vi "Camera Dialog.vi"(8 "error in":errorcluster, 9 "Set Points":dbl[](array[numeric])=[1.0, 5.0, 1.0, 0.0]) -> (0 "error out":errorcluster, 1 "ROI":T3, 2 "Image Out":T1(plugin-control), 3 "Session out":T2="cam1")   [LabVIEW 2012]
uses:
  <vilib>/vision/driver/NI_Vision_Acquisition_Software.lvlib
  <vilib>/userdefined/High Color/IMAQdx.ctl
panel:
  in  "Tab Control":enum32{"Configure", "Help", "Advanced"}(tab)
  in  "Record images":bool
  out "Interface elevation":dbl
  in  "Image folder":path
  in  "Image Save Rate (s)":dbl=10.0 format="%#_5f"
  in  "Update Camera":bool
  in  "Camera Attributes In":string
  out "Camera Attributes":string
  out "Camera error out":errorcluster
  out "stop":bool
  in  "Cancel Button":bool
  in  "OK Button":bool
  # "Use the rectangle tool to define the region of interest where the floc water interface will appear.\nThe region of interest is saved in a configuration file.\n\nChoose a folder to save images during the experiment."
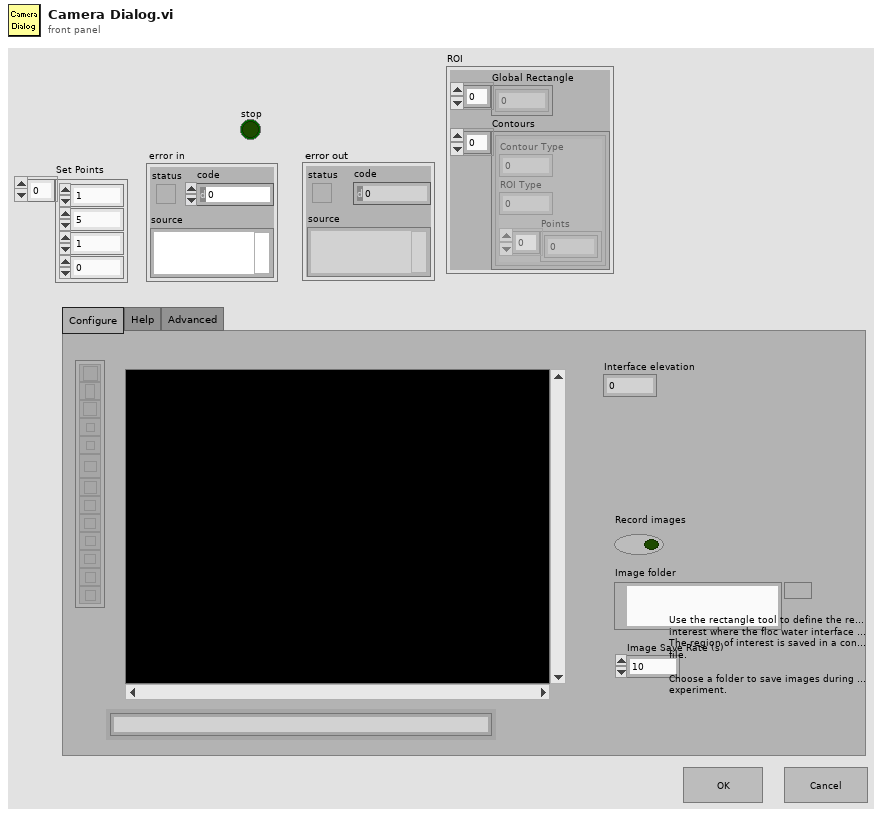
[diagram p1: front panel]
types:
  T1 = typedef "IMAQ Image.ctl" = refnum<image>
  T2 = typedef "IMAQdx.ctl" = refnum<k21>
  T3 = cluster{"Global Rectangle":i32[], "Contours":cluster{"Contour Type":u32, "ROI Type":u32, "Points":i32[]}[]}
  T4 = typedef "Image Type" = u32
  T5 = cluster{"Set Points[0]":dbl, "Set Points[1]":dbl, "Set Points[2]":dbl, "Set Points[3]":dbl}
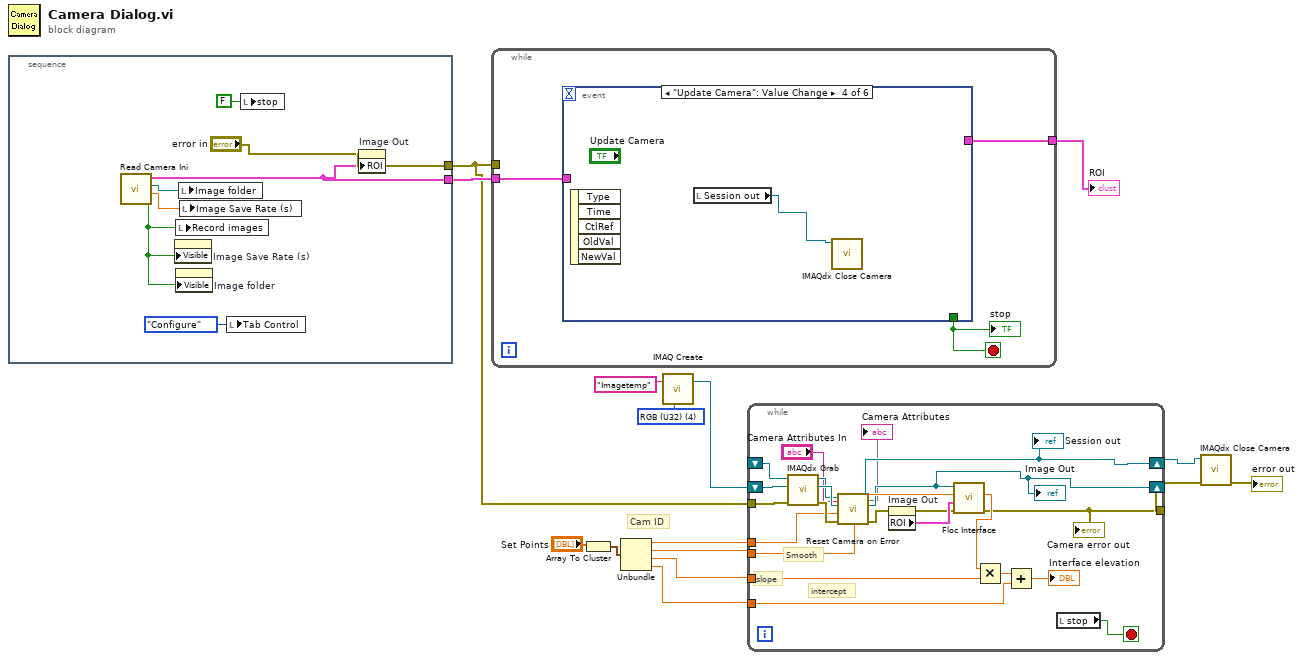
[diagram p0: block diagram]
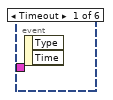
[diagram p2: hidden frame]
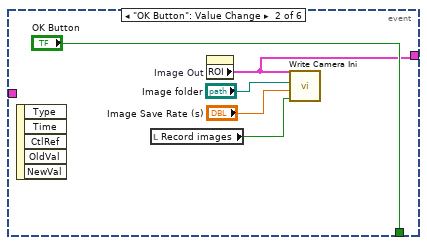
[diagram p3: hidden frame]
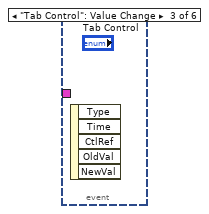
[diagram p4: hidden frame]
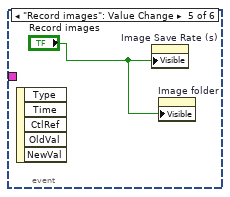
[diagram p5: hidden frame]
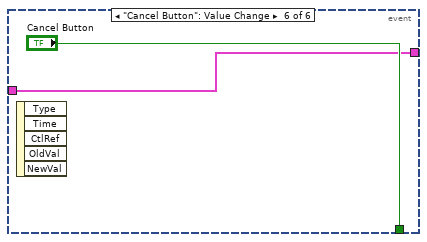
[diagram p6: hidden frame]
diagram:
  w8 = T4 4 items=["Grayscale (U8)", "Grayscale (I16)", "Grayscale (SGL)", "Complex (CSG)", "RGB (U32)", "HSL (U32)", "RGB (U64)", "Grayscale (U16)"] ("Image Type")
  # "Cam ID"
  n1 = stacked-sequence {
    tunnel: [w23] -> w1
    tunnel: [w21] -> w9
    frame #0 {
      n2 = call "Read Camera Ini.vi"() -> ("Record images"=w17:bool, "Image Save Rate (s)"=w18:dbl, "Image folder"=w19:path, "ROI"=w21:T3)  [unwired: 8 in]
      n3 = property on="Image Save Rate (s)" class="DigNum (strict)"("Visible"=w17) -> ()  [unwired: 2 in, 2 out]
      n4 = local write "Record images"(w17) -> ()
      n5 = property on="Image folder" class="Path"("Visible"=w17) -> ()  [unwired: 2 in, 2 out]
      n6 = local write "Image folder"(w19) -> ()
      n7 = local write "Image Save Rate (s)"(w18) -> ()
      n8 = local write "Tab Control"(enum32{"Configure", "Help"}."Configure" ("Tab Control")) -> ()
      n9 = local write "stop"(FALSE ("stop")) -> ()
      n10 = property on="Image Out" class="ImageControl"(error in="error in", "ROI"=w21) -> (error out=w23:errorcluster)  [unwired: 1 in, 1 out]
    }
  }
  n11 = while {
    tunnel: w1 -> [_]
    tunnel: [w25] -> w10
    tunnel: w9 -> [w24]
    stop <- w26 stop-if-true
    n12 = event shown="[3] \"Update Camera\": Value Change" {
      selector: _ -> [_ _ _ _ _ _]
      dyn-events: _ -> [_ _ _ _ _ _]
      timeout: _ -> [_ _ _ _ _ _]
      tunnel: [_ "OK Button" _ _ _ "Cancel Button"] -> w26
      tunnel: [_ w30 _ _ _ w34] -> w25
      tunnel: w24 -> [_ _ _ _ _ w34]
      event Timeout {
        n13 = event-data() -> ()  [unwired: 1 in, 2 out]
      }
      event "OK Button": Value Change {
        n14 = event-data() -> ()  [unwired: 1 in, 5 out]
        n15 = local read "Record images"() -> (w27:bool)
        n16 = property on="Image Out" class="ImageControl"() -> ("ROI"=w30:T3)  [unwired: 2 in, 2 out]
        n17 = call "Write Camera Ini.vi"("Record images"=w27, "Image Save Rate (s)"="Image Save Rate (s)", "Image folder"="Image folder", "ROI"=w30) -> ()  [unwired: 8 in]
      }
      event "Tab Control": Value Change {
        n18 = event-data() -> ()  [unwired: 1 in, 5 out]
      }
      event "Update Camera": Value Change {
        n19 = event-data() -> ()  [unwired: 1 in, 5 out]
        n20 = local read "Session out"() -> (w32:T2)
        n21 = call <vilib>:"IMAQdx Close Camera.vi"("Session In"=w32) -> ()  [unwired: 10 in, 1 out]
      }
      event "Record images": Value Change {
        n22 = event-data() -> ()  [unwired: 1 in, 5 out]
        n23 = property on="Image Save Rate (s)" class="DigNum (strict)"("Visible"="Record images") -> ()  [unwired: 2 in, 2 out]
        n24 = property on="Image folder" class="Path"("Visible"="Record images") -> ()  [unwired: 2 in, 2 out]
      }
      event "Cancel Button": Value Change {
        n25 = event-data() -> ()  [unwired: 1 in, 5 out]
      }
    }
    "stop" <- w26
  }
  "ROI" <- w10
  n26 = Array To Cluster(array="Set Points") -> (cluster=w15:T5)
  n27 = Unbundle(w15) -> ("Set Points[0]"=w3:dbl, "Set Points[1]"=w13:dbl, "Set Points[2]"=w12:dbl, "Set Points[3]"=w11:dbl)
  n28 = call "IMAQ Create"("Image Name"="Imagetemp", "Image Type"=w8) -> ("New Image"=w6:T1)  [unwired: 2 in, 2 out]
  n29 = while {
    tunnel: w1 -> [w56]
    tunnel: w13 -> [w50]
    tunnel: w12 -> [w49]
    tunnel: w11 -> [w48]
    tunnel: [w46] -> w5
    tunnel: w3 -> [w43]
    shift-right: [w39] -> _
    shift-left: w6 -> [w57]
    shift-right: [w38] -> w2
    shift-left: _ -> [w40]
    stop <- w47 stop-if-true
    # "intercept"
    # "slope"
    # "Smooth"
    n30 = call <vilib>:"IMAQdx Grab.vi"("error in"=w56, "Image In"=w57, "Session In"=w40) -> ("error out"=w45:errorcluster, "Image Out"=w42:T1, "Session Out"=w41:T2)  [unwired: 5 in, 1 out]
    n31 = call "Reset Camera on Error.vi"(7:"Camera Attributes In", "error in"=w45, 9:w43, "Image in"=w42, "Session in"=w41) -> ("error out"=w44:errorcluster, "Image out"=w39:T1, "Session out"=w38:T2, 5:→"Camera Attributes")  [unwired: 3 in]
    "Image Out" <- w39
    "Session out" <- w38
    n32 = property on="Image Out" class="ImageControl"(error in=w44) -> (error out=w51:errorcluster, "ROI"=w52:T3)  [unwired: 1 in, 1 out]
    n33 = call "Floc Interface.vi"("error in"=w51, "ROI"=w52, "Interface inputs"=w50, "Image"=w39) -> ("error out"=w46:errorcluster, "Interface elevation"=w55:dbl)  [unwired: 4 in, 2 out]
    "Camera error out" <- w46
    n34 = Multiply(x=w55, y=w49) -> (x*y=w54:dbl)
    n35 = Add(x=w54, y=w48) -> (x+y=→"Interface elevation":dbl)
    n36 = local read "stop"() -> (w47:bool)
  }
  n37 = call <vilib>:"IMAQdx Close Camera.vi"("error in"=w5, "Session In"=w2) -> ("error out"=→"error out":errorcluster)  [unwired: 9 in]
